vi "Test Get Attribute STRING_1.vi"(11 "Test Case In":refnum<class "My Config from XML.lvclass">) -> (0 "error out":errorcluster, 3 "Test Case Out":refnum<class "My Config from XML.lvclass">)   [LabVIEW 2024, in "My Config from XML.lvclass"]
uses:
  My Config from XML.lvclass
  My Config from XML.lvclass/My Config from XML.ctl
  4993e8ee-a06a-463a-9684-69129f64d5ce.vi
  Config from XML/Config from XML.lvclass
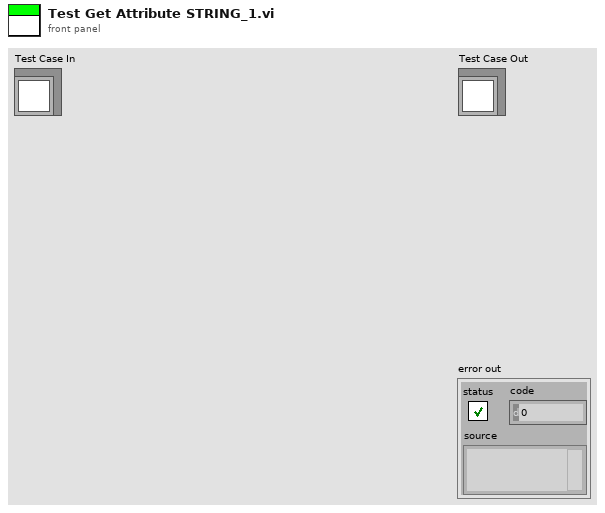
[diagram p1: front panel]
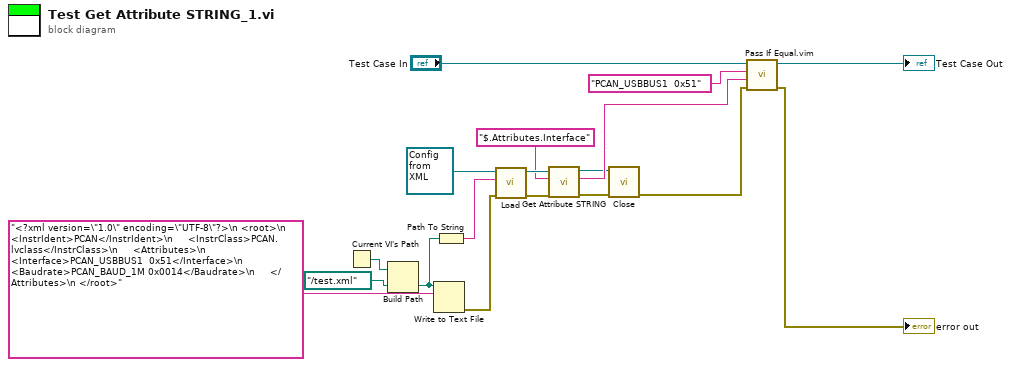
[diagram p0: block diagram]
diagram:
  n1 = Current VI's Path() -> (path=w12:path)
  n2 = Build Path(base path=w12, name or relative path=path "../test.xml") -> (appended path=w10:path)
  n3 = Write to Text File(file (use dialog)=w10, text="<?xml version=\"1.0\" encoding=\"UTF-8\"?>\n <root>\n     <InstrIdent>PCAN</InstrIdent>\n     <InstrClass>PCAN.lvclass</InstrClass>\n     <Attributes>\n         <Interface>PCAN_USBBUS1  0x51</Interface>\n         <Baudrate>PCAN_BAUD_1M 0x0014</Baudrate>\n     </Attributes>\n </root>") -> (error out=w8:errorcluster)  [unwired: 2 in, 2 out]
  n4 = Path To String(path=w10) -> (string=w9:string)
  n5 = call-dynamic "Load.vi"("error in"=w8, "Source"=w9, "Config from XML in"=refnum<class "Config from XML.lvclass"> refnum ("Config from XML.lvclass")) -> ("error out"=w6:errorcluster, "Config from XML out"=w7:refnum<class "Config from XML.lvclass">)  [unwired: 7 in]
  n6 = call-dynamic "Get Attribute STRING.vi"("error in"=w6, "Attribute"="$.Attributes.Interface", "Config from XML in"=w7) -> ("error out"=w2:errorcluster, "Value"=w4:string, "Config from XML out"=w3:refnum<class "Config from XML.lvclass">)  [unwired: 6 in]
  n7 = call-dynamic "Close.vi"("error in"=w2, "Config from XML in"=w3) -> ("error out"=w1:errorcluster)  [unwired: 8 in, 1 out]
  n8 = call "Pass If Equal.vim"("error in (no error)"=w1, "Actual"=w4, "Expected"="PCAN_USBBUS1  0x51", "LUnit Test Case In"="Test Case In") -> ("error out"=→"error out":errorcluster, "LUnit Test Case Out"=→"Test Case Out":refnum<class "My Config from XML.lvclass">)  [unwired: 6 in]
